vi "config UI to not UI (AO and AI).vi"(11 "New Ch []":T1 {"AI terminal config" items=[""=-1, "differential"=10106, "pseudodifferential"=12529]; "AI.Coupling" items=[""=0, "AC"=10045, "DC"=10050, "GND"=10066]; "AO terminal config" items=[""=-1, "differential"=10106, "pseudodifferential"=12529]}) -> (2 "AO Config":T7 {"terminal configuration" items=[""=-1, "differential"=10106, "pseudodifferential"=12529]}, 3 "AI Config":T9 {"terminal configuration" items=[""=-1, "differential"=10106, "pseudodifferential"=12529]; "Coupling" items=[""=0, "AC"=10045, "DC"=10050, "GND"=10066]})   [LabVIEW 2019, in "Instrument.Lockin.lvlib" / "Instrument.Lockin.lvclass"]
uses:
  Instrument.Lockin.lvclass
  Instrument.DAQ/Typedefs/DAQ.Config.AI--Cluster--Array.ctl
  Instrument.DAQ/Typedefs/DAQ.Config.AI.Coupling--enum.ctl
  Instrument.DAQ/Typedefs/DAQ.Config.AI.Range--enum.ctl
  Instrument.DAQ/Typedefs/DAQ.TerminalConfiguration--ring.ctl
  Instrument.DAQ/Typedefs/DAQ.Type--enum.ctl
  Instrument.DAQ/Typedefs/DAQ.Config.AO--Cluster--Array.ctl
  Instrument.DAQ/Typedefs/DAQ.Config.AO.Range--enum.ctl
  Instrument.DAQ/Typedefs/DAQ.Configuration--Cluster--Array.ctl
  Instrument.DAQ/Typedefs/DAQ.Configuration--Cluster.ctl
  Instrument.DAQ/Instrument.DAQ.lvclass
panel:
  # "Device"
  # "AI.Ch"
  # "AI.Range"
  # "AI.Coupling"
  # "AO.Ch"
  # "AO.Range"
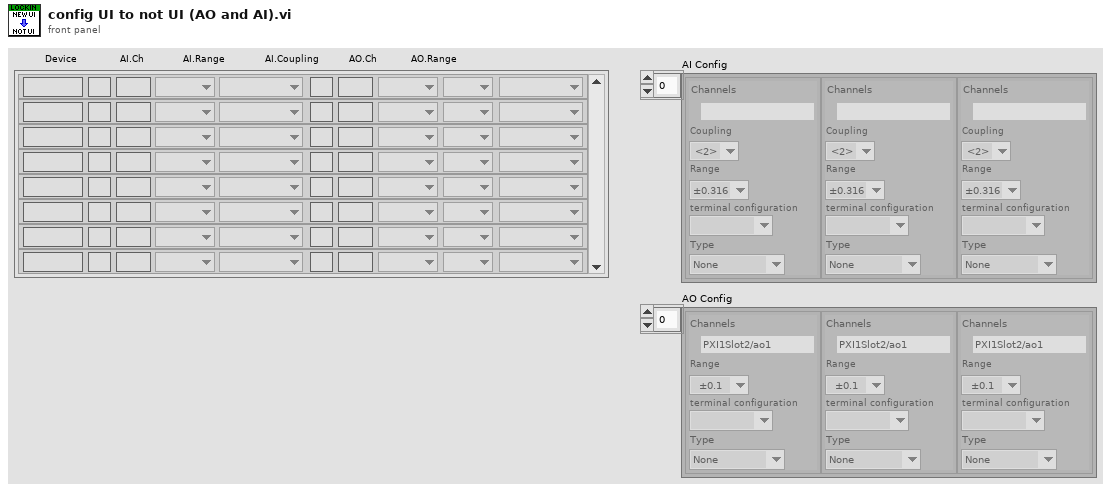
[diagram p1: front panel]
types:
  T1 = typedef "Instrument.Lockin.lvlib/Instrument.DAQ.lvclass/DAQ.Configuration--Cluster--Array.ctl" = T2[]
  T2 = typedef "Instrument.Lockin.lvlib/Instrument.DAQ.lvclass/DAQ.Configuration--Cluster.ctl" = cluster{"Device":string, "Lockin.AO":string, "AO.Ch":string, "AO.Range":T3, "AO terminal config":T4, "Lockin.AI":string, "AI.Ch":string, "AI.Range":T5, "AI.Coupling":T6, "AI terminal config":T4}
  T3 = typedef "Instrument.Lockin.lvlib/Instrument.DAQ.lvclass/DAQ.Config.AO.Range--enum.ctl" = enum16{"±0.1", "±1.0", "±10.0", ""}
  T4 = typedef "Instrument.Lockin.lvlib/Instrument.DAQ.lvclass/DAQ.TerminalConfiguration--ring.ctl" = i32
  T5 = typedef "Instrument.Lockin.lvlib/Instrument.DAQ.lvclass/DAQ.Config.AI.Range--enum.ctl" = enum16{"±0.316", "±1.00", "±3.16", "±10.0", "±31.6", "±42.4", ""}
  T6 = typedef "Instrument.Lockin.lvlib/Instrument.DAQ.lvclass/DAQ.Config.AI.Coupling--enum.ctl" = u16
  T7 = typedef "Instrument.Lockin.lvlib/Instrument.DAQ.lvclass/DAQ.Config.AO--Cluster--Array.ctl" = cluster{"Channels":tag, "Range":T3, "terminal configuration":T4, "Type":T8}[]
  T8 = typedef "Instrument.Lockin.lvlib/Instrument.DAQ.lvclass/DAQ.Type--enum.ctl" = enum16{"None", "USB-4431", "PXI-446x"}
  T9 = typedef "Instrument.Lockin.lvlib/Instrument.DAQ.lvclass/DAQ.Config.AI--Cluster--Array.ctl" = cluster{"Channels":tag, "Coupling":T6, "Range":T5, "terminal configuration":T4, "Type":T8}[]
  T10 = cluster{"Channels":tag, "Range":T3, "terminal configuration":T4, "Type":T8}
  T11 = cluster{"Channels":tag, "Coupling":T6, "Range":T5, "terminal configuration":T4, "Type":T8}
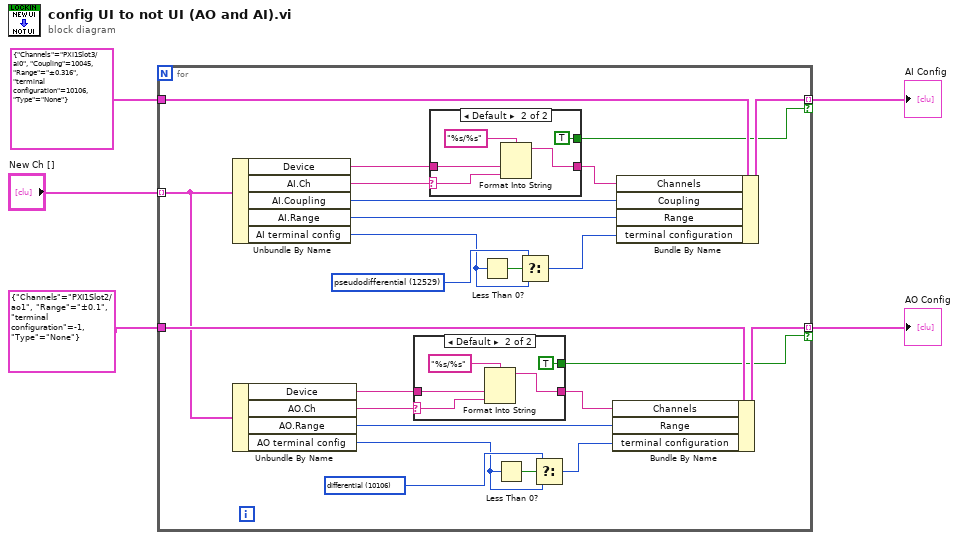
[diagram p0: block diagram]
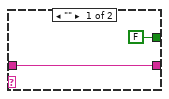
[diagram p2: hidden frame]
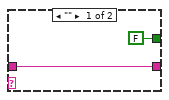
[diagram p3: hidden frame]
diagram:
  n1 = for {
    tunnel: T11 {"Channels"="PXI1Slot3/ai0", "Coupling"=10045, "Range"=enum."±0.316", "terminal configuration"=10106, "Type"=enum."None"} ("Config.AI") -> [w29]
    tunnel: "New Ch []" -> [w15] mode=indexing
    tunnel: [w26] -> w5 mode=indexing if=w19
    tunnel: T10 {"Channels"="PXI1Slot2/ao1", "Range"=enum."±0.1", "terminal configuration"=-1, "Type"=enum."None"} ("Config.AO") -> [w25]
    tunnel: [w24] -> w3 mode=indexing if=w16
    w12 = T4 10106 items=[""=-1, "differential"=10106, "pseudodifferential"=12529] ("terminal configuration")
    w13 = T4 12529 items=[""=-1, "differential"=10106, "pseudodifferential"=12529] ("terminal configuration")
    n2 = Unbundle By Name(w15) -> ("Device"=w23:string, "AI.Ch"=w20:string, "AI.Coupling"=w28:T6, "AI.Range"=w27:T5, "AI terminal config"=w9:T4)
    n3 = Unbundle By Name(w15) -> ("Device"=w18:string, "AO.Ch"=w6:string, "AO.Range"=w22:T3, "AO terminal config"=w10:T4)
    n4 = case shown="Default" w6 {
      selector: w6 -> [_ w33]
      tunnel: w18 -> [w31 w35]
      tunnel: [w31 w34] -> w17
      tunnel: [FALSE TRUE] -> w16
      frame "" {
      }
      frame Default {
        n5 = Format Into String(format string="%s/%s", w35, w33) -> (resulting string=w34:string)  [unwired: 2 in, 1 out]
      }
    }
    n6 = case shown="Default" w20 {
      selector: w20 -> [_ w40]
      tunnel: w23 -> [w38 w42]
      tunnel: [w38 w41] -> w21
      tunnel: [FALSE TRUE] -> w19
      frame "" {
      }
      frame Default {
        n7 = Format Into String(format string="%s/%s", w42, w40) -> (resulting string=w41:string)  [unwired: 2 in, 1 out]
      }
    }
    n8 = Less Than 0?(x=w9) -> (x < 0?=w14:bool)
    n9 = Less Than 0?(x=w10) -> (x < 0?=w11:bool)
    n10 = Select(t=w13, s=w14, f=w9) -> (s? t:f=w8:T4)
    n11 = Select(t=w12, s=w11, f=w10) -> (s? t:f=w7:T4)
    n12 = Bundle By Name(cluster=w25, "Channels"=w17, "Range"=w22, "terminal configuration"=w7) -> (w24:T10)
    n13 = Bundle By Name(cluster=w29, "Channels"=w21, "Coupling"=w28, "Range"=w27, "terminal configuration"=w8) -> (w26:T11)
  }
  "AI Config" <- w5
  "AO Config" <- w3
